vi "Send Active DUT SMS.vi"(8 "error in (no error)":errorcluster, 10 "SIM Slot (1)":i32=1, 11 "VISA resource name":refnum<visa-resource-name>) -> (0 "error out":errorcluster, 3 "VISA resource name out":refnum<visa-resource-name>)   [LabVIEW 2020, in "Rohde&Schwarz CMXP Base.lvlib"]
doc: "Sends an SMS with default text to a default number.\n\nAttributes:\nRSCMXPBASE_ATTR_SELECT_ACTIVE_DUT_SIM_SLOT\nRSCMXPBASE_ATTR_ACTIVE_DUT_SMS_SEND\n\nRemote-control command:\nPROCedure:DUT:MODem<ModemIdx>:CONTrol:SMS"
uses:
  <instrlib>/Rohde&Schwarz CMXP Base/Rohde&Schwarz CMXP Base.lvlib
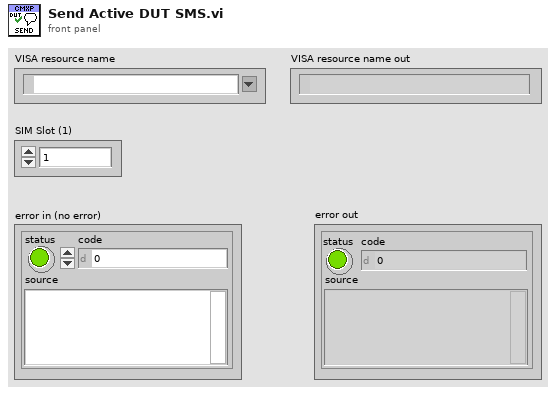
[diagram p1: front panel]
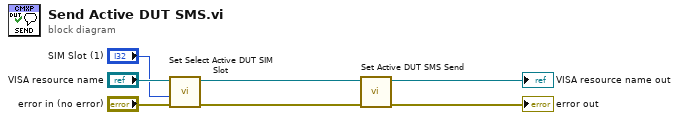
[diagram p0: block diagram]
diagram:
  n1 = call "Set Select Active DUT SIM Slot"("error in (no error)"="error in (no error)", "Select Active DUT SIM Slot (0)"="SIM Slot (1)", "instrument handle"="VISA resource name") -> ("error out"=w5:errorcluster, "instrument handle out"=w4:refnum<visa-resource-name>)  [unwired: 7 in]
  n2 = call "Set Active DUT SMS Send"("error in (no error)"=w5, "instrument handle"=w4) -> ("error out"=→"error out":errorcluster, "instrument handle out"=→"VISA resource name out":refnum<visa-resource-name>)  [unwired: 8 in]
